vi "Escritura_BaseDatos.vi"() -> ()   [LabVIEW 2020]
uses:
  <vilib>/httpClient/PUTBuffer.vi
  <vilib>/httpClient/LabVIEWHTTPClient.lvlib
panel:
  in  "Accionamiento [mA]":dbl(knob) scale=0.0..10.0
  in  "Rele":bool
  in  "stop":bool
  out "headers":string
  out "body":string
  out "error out":errorcluster
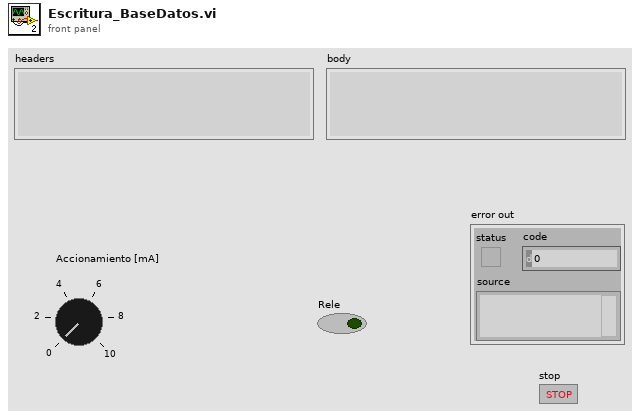
[diagram p1: front panel]
types:
  T1 = cluster{"Accionamiento":dbl, "Data":string, "Hora":string, "Rele":bool}
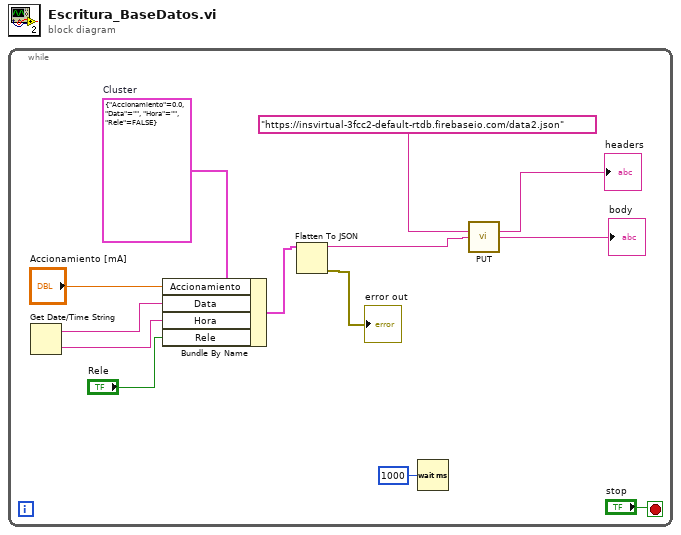
[diagram p0: block diagram]
diagram:
  n1 = while {
    stop <- "stop" stop-if-true
    w7 = T1 {"Accionamiento"=0.0, "Data"="", "Hora"="", "Rele"=FALSE}  # Cluster
    n2 = Get Date/Time String() -> (date string=w2:string, time string=w1:string)  [unwired: 3 in]
    n3 = Bundle By Name(cluster=w7, "Accionamiento"="Accionamiento [mA]", "Data"=w2, "Hora"=w1, "Rele"="Rele") -> (w6:T1)
    n4 = Flatten To JSON(anything=w6) -> (JSON string=w5:string, 11:→"error out":errorcluster)  [unwired: 2 in]
    n5 = Wait (ms)(milliseconds to wait=u32 1000) -> ()  [unwired: 1 out]
    n6 = call-poly <vilib>:"PUT.vi"("url"="https://insvirtual-3fcc2-default-rtdb.firebaseio.com/data2.json", "buffer"=w5) -> ("headers"=→"headers":string, "body"=→"body":string)  [unwired: 10 in, 2 out]
  }
